vi "Basic RT Test.vi"   [LabVIEW 2016]
uses:
  Utilities/FPGA Interface/FPGA Interface.lvclass
  Remote Terminal/TypeDefs/Command Type.ctl
  1553 SubComponent/TypeDefs/Parameter Table Data.ctl
  1553 SubComponent/TypeDefs/Scaling Information.ctl
  Remote Terminal/TypeDefs/RT Configuration.ctl
  Remote Terminal/TypeDefs/Command Configuration.ctl
  Remote Terminal/Remote Terminal.lvclass
  D:/SVN/Products/BCI-1553/Software/Development/2016/RealTime/1553 SubComponent/1553 SubComponent.lvclass
  1553 Component/1553 Component.lvclass
  1553 SubComponent/1553 SubComponent.lvclass
types:
  T1 = typedef "BCI-1553 API.lvlib/1553 SubComponent.lvclass/Parameter Table Data.ctl" = cluster{"Parameter Name":string, "Base Word":u16, "Address":u16, "Value":u64, "Mask":u16[], "Scaling Info":T2}
  T2 = typedef "BCI-1553 API.lvlib/1553 SubComponent.lvclass/Scaling Information.ctl" = cluster{"Bit Offset":i32, "Bit Count":i32, "LSB Resolution":dbl, "2's Complement":bool, "Big Endian":bool, "Sign Bit":bool}
  T3 = typedef "BCI-1553 API.lvlib/Remote Terminal.lvclass/Command Type.ctl" = enum16{"Transmit", "Receive", "Mode Code Tx", "Mode Code Rx"}
  T4 = typedef "BCI-1553 API.lvlib/Remote Terminal.lvclass/Command Configuration.ctl" = cluster{"Command Type":T3, "Mode Code ID (1-32)":u16, "SubAddress (1-30)":u16, "Word Count (1-32)":u16, "Illegal Command":bool, "Broadcast":bool, "Data":u16[], "Data Fields":T1[]}
  T5 = typedef "BCI-1553 API.lvlib/Remote Terminal.lvclass/RT Configuration.ctl" = cluster{"RT-RT TimeOut (us)":u8, "Inhibit Bus A":bool, "Inhibit Bus B":bool, "Broadcast CMD Invalid":bool, "UnDef MCs Invalid":bool, "Notice 2 Data Storage":bool, "SMCP":bool, "Temp RX Buffer":bool, "Alt BIT Enable":bool, "Auto Bus Shutdown":bool, "MC 17 Sync":u8, "MC 16 SR Reset":bool, "MC 8 Reset":bool}
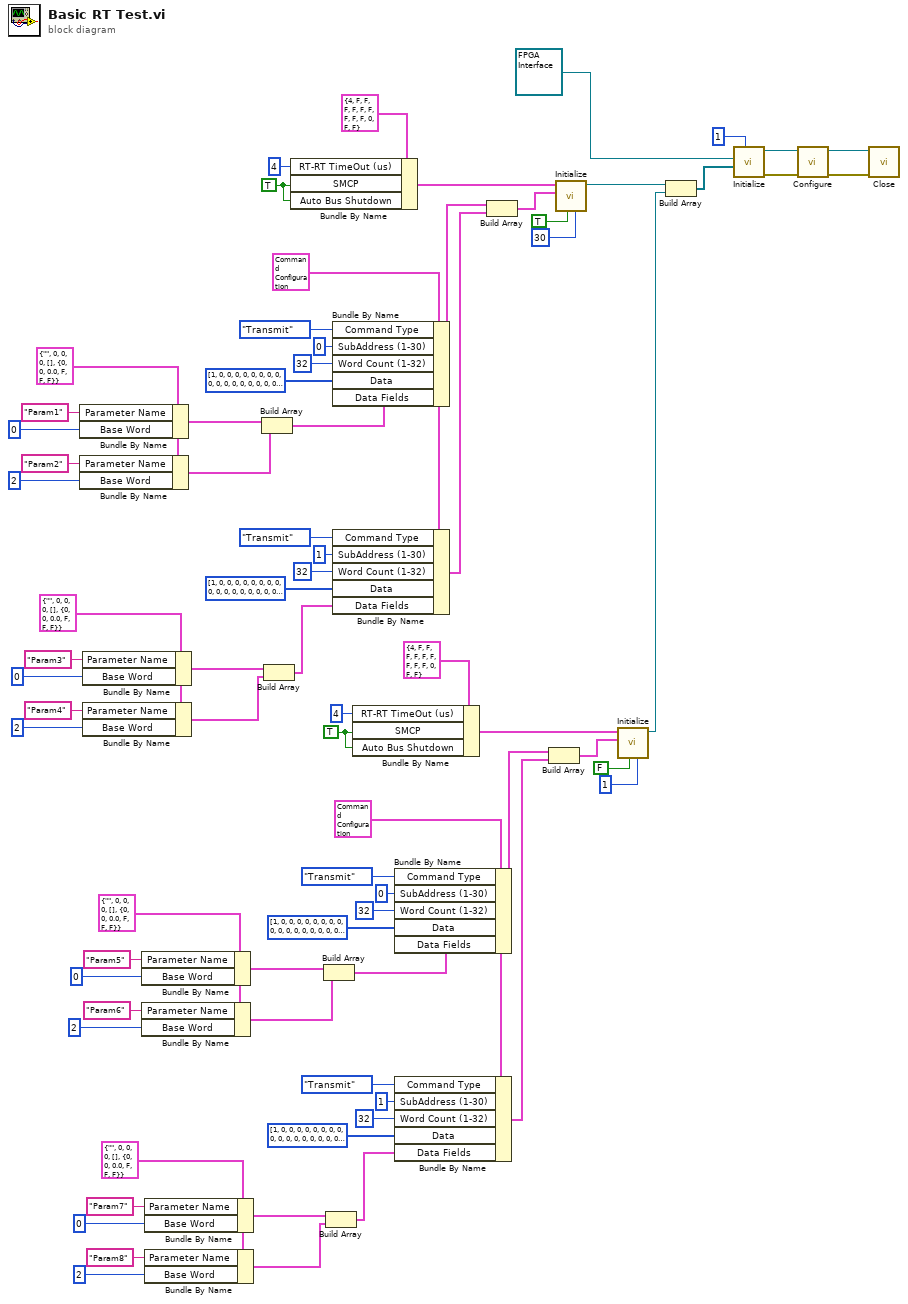
[diagram p0: block diagram]
diagram:
  w32 = T1 {"Parameter Name"="", "Base Word"=0, "Address"=0, "Value"=0, "Mask"=[], "Scaling Info"={"Bit Offset"=0, "Bit Count"=0, "LSB Resolution"=0.0, "2's Complement"=FALSE, "Big Endian"=FALSE, "Sign Bit"=FALSE}} ("Parameter Table Data")
  w21 = T1 {"Parameter Name"="", "Base Word"=0, "Address"=0, "Value"=0, "Mask"=[], "Scaling Info"={"Bit Offset"=0, "Bit Count"=0, "LSB Resolution"=0.0, "2's Complement"=FALSE, "Big Endian"=FALSE, "Sign Bit"=FALSE}} ("Parameter Table Data")
  w26 = T4 {"Command Type"=enum."Transmit", "Mode Code ID (1-32)"=0, "SubAddress (1-30)"=1, "Word Count (1-32)"=32, "Illegal Command"=FALSE, "Broadcast"=FALSE, "Data"=[1, 0, 0, 0, 0, 0, 0, 0, 0, 0, 0, 0, 0, 0, 0, 0, 0, 0, 0, 0, 43690, 0, 0, 0, 0, 0, 0, 0, 0, 0, 0, 65535], "Data Fields"=[{"Parameter Name"="P1", "Base Word"=0, "Address"=0, "Value"=0, "Mask"=[], "Scaling Info"={"Bit Offset"=0, "Bit Count"=0, "LSB Resolution"=0.0, "2's Complement"=FALSE, "Big Endian"=FALSE, "Sign Bit"=FALSE}}]} ("CMD Configuration")
  w8 = TRUE ("SMCP")
  w39 = T1 {"Parameter Name"="", "Base Word"=0, "Address"=0, "Value"=0, "Mask"=[], "Scaling Info"={"Bit Offset"=0, "Bit Count"=0, "LSB Resolution"=0.0, "2's Complement"=FALSE, "Big Endian"=FALSE, "Sign Bit"=FALSE}} ("Parameter Table Data")
  w50 = T1 {"Parameter Name"="", "Base Word"=0, "Address"=0, "Value"=0, "Mask"=[], "Scaling Info"={"Bit Offset"=0, "Bit Count"=0, "LSB Resolution"=0.0, "2's Complement"=FALSE, "Big Endian"=FALSE, "Sign Bit"=FALSE}} ("Parameter Table Data")
  w45 = T4 {"Command Type"=enum."Transmit", "Mode Code ID (1-32)"=0, "SubAddress (1-30)"=1, "Word Count (1-32)"=32, "Illegal Command"=FALSE, "Broadcast"=FALSE, "Data"=[1, 0, 0, 0, 0, 0, 0, 0, 0, 0, 0, 0, 0, 0, 0, 0, 0, 0, 0, 0, 43690, 0, 0, 0, 0, 0, 0, 0, 0, 0, 0, 65535], "Data Fields"=[{"Parameter Name"="P1", "Base Word"=0, "Address"=0, "Value"=0, "Mask"=[], "Scaling Info"={"Bit Offset"=0, "Bit Count"=0, "LSB Resolution"=0.0, "2's Complement"=FALSE, "Big Endian"=FALSE, "Sign Bit"=FALSE}}]} ("CMD Configuration")
  w73 = TRUE ("SMCP")
  n1 = Bundle By Name(cluster=w50, "Parameter Name"="Param1", "Base Word"=u16 0) -> (w60:T1)
  n2 = Bundle By Name(cluster=w50, "Parameter Name"="Param2", "Base Word"=u16 2) -> (w59:T1)
  n3 = Bundle By Name(cluster=w39, "Parameter Name"="Param3", "Base Word"=u16 0) -> (w38:T1)
  n4 = Bundle By Name(cluster=w39, "Parameter Name"="Param4", "Base Word"=u16 2) -> (w37:T1)
  n5 = Bundle By Name(cluster=w21, "Parameter Name"="Param5", "Base Word"=u16 0) -> (w19:T1)
  n6 = Bundle By Name(cluster=w21, "Parameter Name"="Param6", "Base Word"=u16 2) -> (w20:T1)
  n7 = Bundle By Name(cluster=w32, "Parameter Name"="Param7", "Base Word"=u16 0) -> (w33:T1)
  n8 = Bundle By Name(cluster=w32, "Parameter Name"="Param8", "Base Word"=u16 2) -> (w34:T1)
  n9 = Build Array(w60, w59) -> (w61:T1[])
  n10 = Build Array(w38, w37) -> (w36:T1[])
  n11 = Bundle By Name(cluster=T5 {"RT-RT TimeOut (us)"=4, "Inhibit Bus A"=FALSE, "Inhibit Bus B"=FALSE, "Broadcast CMD Invalid"=FALSE, "UnDef MCs Invalid"=FALSE, "Notice 2 Data Storage"=FALSE, "SMCP"=FALSE, "Temp RX Buffer"=FALSE, "Alt BIT Enable"=FALSE, "Auto Bus Shutdown"=FALSE, "MC 17 Sync"=0, "MC 16 SR Reset"=FALSE, "MC 8 Reset"=FALSE} ("RT Configuration"), "RT-RT TimeOut (us)"=u8 4, "SMCP"=w73, "Auto Bus Shutdown"=w73) -> (w72:T5)
  n12 = Build Array(w19, w20) -> (w18:T1[])
  n13 = Build Array(w33, w34) -> (w35:T1[])
  n14 = Bundle By Name(cluster=w45, "Command Type"=Command_Type."Transmit", "SubAddress (1-30)"=u16 0, "Word Count (1-32)"=u16 32, "Data"=u16[] [1, 0, 0, 0, 0, 0, 0, 0, 0, 0, 0, 0, 0, 0, 0, 0, 0, 0, 0, 0, 0, 0, 0, 0, 0, 0, 0, 0, 0, 0, 0, 65535], "Data Fields"=w61) -> (w68:T4)
  n15 = Bundle By Name(cluster=w45, "Command Type"=Command_Type."Transmit", "SubAddress (1-30)"=u16 1, "Word Count (1-32)"=u16 32, "Data"=u16[] [1, 0, 0, 0, 0, 0, 0, 0, 0, 0, 0, 0, 0, 0, 0, 0, 0, 0, 0, 0, 0, 0, 0, 0, 0, 0, 0, 0, 0, 0, 0, 65535], "Data Fields"=w36) -> (w44:T4)
  n16 = Bundle By Name(cluster=T5 {"RT-RT TimeOut (us)"=4, "Inhibit Bus A"=FALSE, "Inhibit Bus B"=FALSE, "Broadcast CMD Invalid"=FALSE, "UnDef MCs Invalid"=FALSE, "Notice 2 Data Storage"=FALSE, "SMCP"=FALSE, "Temp RX Buffer"=FALSE, "Alt BIT Enable"=FALSE, "Auto Bus Shutdown"=FALSE, "MC 17 Sync"=0, "MC 16 SR Reset"=FALSE, "MC 8 Reset"=FALSE} ("RT Configuration"), "RT-RT TimeOut (us)"=u8 4, "SMCP"=w8, "Auto Bus Shutdown"=w8) -> (w9:T5)
  n17 = Bundle By Name(cluster=w26, "Command Type"=Command_Type."Transmit", "SubAddress (1-30)"=u16 0, "Word Count (1-32)"=u16 32, "Data"=u16[] [1, 0, 0, 0, 0, 0, 0, 0, 0, 0, 0, 0, 0, 0, 0, 0, 0, 0, 0, 0, 0, 0, 0, 0, 0, 0, 0, 0, 0, 0, 0, 65535], "Data Fields"=w18) -> (w13:T4)
  n18 = Bundle By Name(cluster=w26, "Command Type"=Command_Type."Transmit", "SubAddress (1-30)"=u16 1, "Word Count (1-32)"=u16 32, "Data"=u16[] [1, 0, 0, 0, 0, 0, 0, 0, 0, 0, 0, 0, 0, 0, 0, 0, 0, 0, 0, 0, 0, 0, 0, 0, 0, 0, 0, 0, 0, 0, 0, 65535], "Data Fields"=w35) -> (w27:T4)
  n19 = Build Array(w68, w44) -> (w71:T4[])
  n20 = Build Array(w13, w27) -> (w10:T4[])
  n21 = call "Initialize.vi"("RT Address (0-30)"=u8 30, "RT 1?"=TRUE, "Commands"=w71, "RT Configuration"=w72) -> ("Remote Terminal out"=w57:refnum<class "Remote Terminal.lvclass">)  [unwired: 6 in, 1 out]
  n22 = call "Initialize.vi"("RT Address (0-30)"=u8 1, "RT 1?"=FALSE, "Commands"=w10, "RT Configuration"=w9) -> ("Remote Terminal out"=w1:refnum<class "Remote Terminal.lvclass">)  [unwired: 6 in, 1 out]
  n23 = Build Array(w57, w1) -> (w56:refnum<class "Remote Terminal.lvclass">[])
  n24 = call "Initialize.vi"("Component ID (1-8)"=u8 1 ("Component ID"), "SubComponents"=w56, "FPGA Interface"=refnum<class "FPGA Interface.lvclass"> refnum) -> ("error out"=w53:errorcluster, "1553 Component out"=w54:refnum<class "1553 Component.lvclass">)  [unwired: 7 in]
  n25 = call-dynamic "Configure.vi"("error in (no error)"=w53, "1553 Component in"=w54) -> ("error out"=w51:errorcluster, "1553 Component out"=w52:refnum<class "1553 Component.lvclass">)  [unwired: 8 in]
  n26 = call-dynamic "Close.vi"("error in (no error)"=w51, "1553 Component in"=w52) -> ()  [unwired: 9 in, 1 out]
